vi "Update Guest Name.vi"(0 "Hotel Management Tool Model in":refnum<class "Hotel Management Tool Model.lvclass">, 5 "Rooms Manager GUID":string, 7 "IsAvailable":bool, 9 "Guest Name":string, 11 "error in (no error)":errorcluster) -> (4 "Hotel Management Tool Model out":refnum<class "Hotel Management Tool Model.lvclass">, 15 "error out":errorcluster)   [LabVIEW 2023, in "Hotel Management Tool Model.lvlib" / "Hotel Management Tool Model.lvclass"]
uses:
  Hotel Management Tool Model.lvclass
  Hotel Management Tool Model.lvclass/Hotel Management Tool Model.ctl
  Rooms Manager Model/Rooms Manager Model Messages/Update Guest Name Msg/Update Guest Name Msg.lvclass
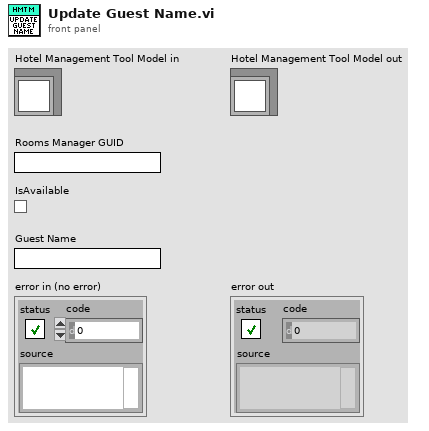
[diagram p1: front panel]
types:
  T1 = map{string, refnum<class "Message Enqueuer.lvclass">}
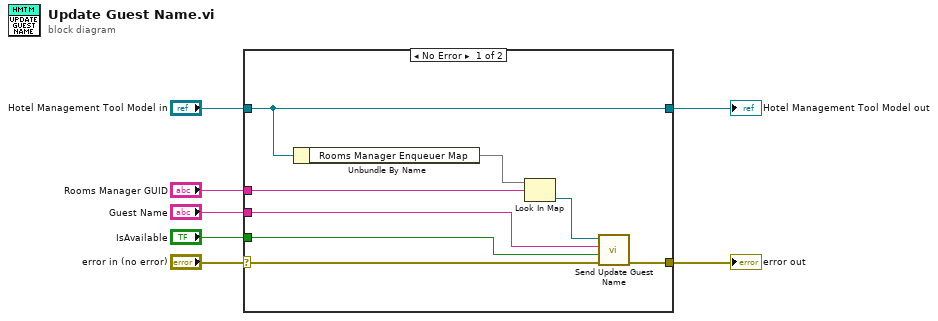
[diagram p0: block diagram]
diagram:
  n1 = case shown="No Error" "error in (no error)" {
    selector: "error in (no error)" -> [w15 w17]
    tunnel: [w14 w17] -> w6
    tunnel: [w13 w16] -> w4
    tunnel: "Hotel Management Tool Model in" -> [w13 w16]
    tunnel: "Rooms Manager GUID" -> [w11 _]
    tunnel: "Guest Name" -> [w9 _]
    tunnel: "IsAvailable" -> [w8 _]
    frame No Error {
      n2 = Unbundle By Name(w13) -> ("Rooms Manager Enqueuer Map"=w12:T1)
      n3 = Look In Map(map=w12, key=w11) -> (value=w10:refnum<class "Message Enqueuer.lvclass">)  [unwired: 1 in, 1 out]
      n4 = call "Send Update Guest Name.vi"("error in (no error)"=w15, "IsAvailable"=w8, "Guest Name"=w9, "Message Enqueuer"=w10) -> ("error out"=w14:errorcluster)  [unwired: 6 in, 1 out]
    }
    frame Error {
    }
  }
  "error out" <- w6
  "Hotel Management Tool Model out" <- w4
